vi "convertToKeyValuePair_boolean.vi"(8 "error in (no error)":errorcluster, 10 "value":bool, 11 "name":string) -> (0 "error out":errorcluster, 3 "string converted":string)   [LabVIEW 2018]
doc: "Convert a boolean into a key value pair as string."
uses:
  convertToKeyValuePair_string.vi
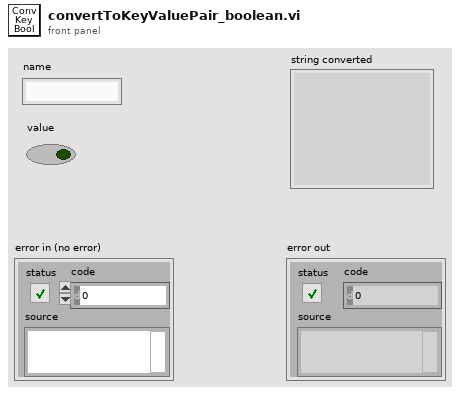
[diagram p1: front panel]
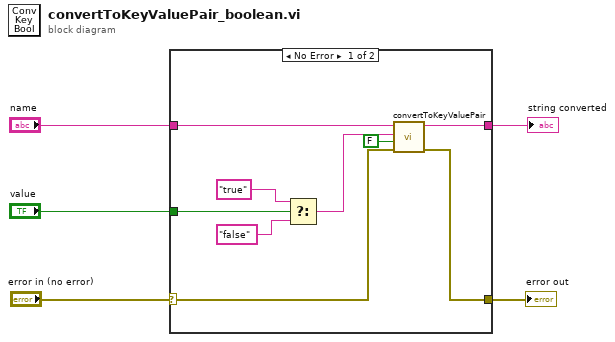
[diagram p0: block diagram]
diagram:
  n1 = case shown="No Error" "error in (no error)" {
    selector: "error in (no error)" -> [w8 w15]
    tunnel: [w10 _] -> w5
    tunnel: "name" -> [w11 _]
    tunnel: [w7 w15] -> w2
    tunnel: "value" -> [w13 _]
    frame No Error {
      n2 = Select(t="true" ("string"), s=w13, f="false" ("string")) -> (s? t:f=w9:string)
      n3 = call-poly "convertToKeyValuePair.vi"("error in (no error)"=w8, "double quotes (T)"=FALSE, "value"=w9, "name"=w11) -> ("error out"=w7:errorcluster, "string converted"=w10:string)  [unwired: 6 in]
    }
    frame Error {
    }
  }
  "error out" <- w2
  "string converted" <- w5
